vi "Bishop_Init.vi"(8 "error in (no error)":errorcluster, 10 "pieceColor":T1, 11 "Object in":refnum<class "Bishop.lvclass">) -> (0 "error out":errorcluster, 3 "object out":refnum<class "Bishop.lvclass">)   [LabVIEW 2020]
uses:
  Bishop.lvclass
  C:/_repos/_personal/Chess/Chess_LV/source/Pieces/Piece.lvclass
  C:/_repos/_personal/Chess/Chess_LV/source/Pieces/Bishop/Bishop.lvclass
  typedefs/pieceColor.ctl
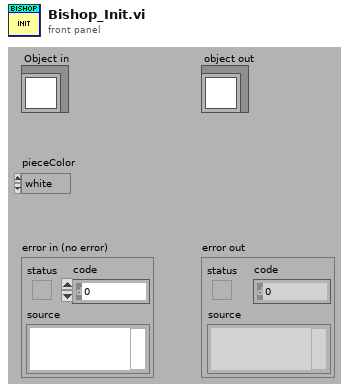
[diagram p1: front panel]
types:
  T1 = typedef "pieceColor.ctl" = enum16{"white", "black"}
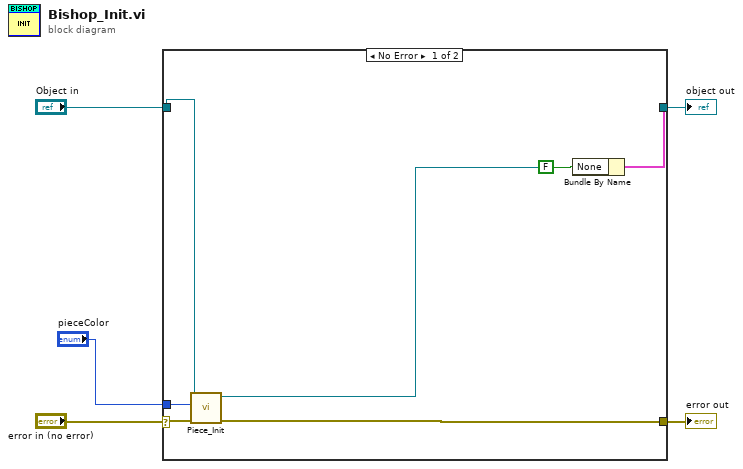
[diagram p0: block diagram]
diagram:
  n1 = case shown="No Error" "error in (no error)" {
    selector: "error in (no error)" -> [w10 w13]
    tunnel: [w12 w14] -> w5
    tunnel: "Object in" -> [w8 w14]
    tunnel: [w9 w13] -> w2
    tunnel: "pieceColor" -> [w6 _]
    frame No Error {
      n2 = call-dynamic "Piece_Init.vi"("error in (no error)"=w10, "pieceColor"=w6, "object in"=w8) -> ("error out"=w9:errorcluster, "object out"=w7:refnum<class "Bishop.lvclass">)  [unwired: 7 in]
      n3 = Bundle By Name(cluster=w7, "None"=FALSE) -> (w12:cluster{})
    }
    frame Error {
    }
  }
  "object out" <- w5
  "error out" <- w2
